vi "HW XML Rx - Write.vi"(0 "String (in)":string, 7 "Parameter Array":T1[](array[typedef])) -> (4 "String (out)":string)   [LabVIEW 2017]
uses:
  Controls/Database_Array.ctl
  Controls/Encoding.ctl
  <userlib>/_OpenG.lib/array/array.llb/Remove Duplicates from 1D Array (I32)__ogtk.vi
  <userlib>/_OpenG.lib/array/array.llb/Filter 1D Array with Scalar (I32)__ogtk.vi
  <userlib>/_OpenG.lib/array/array.llb/Index 1D Array Elements (Variant)__ogtk.vi
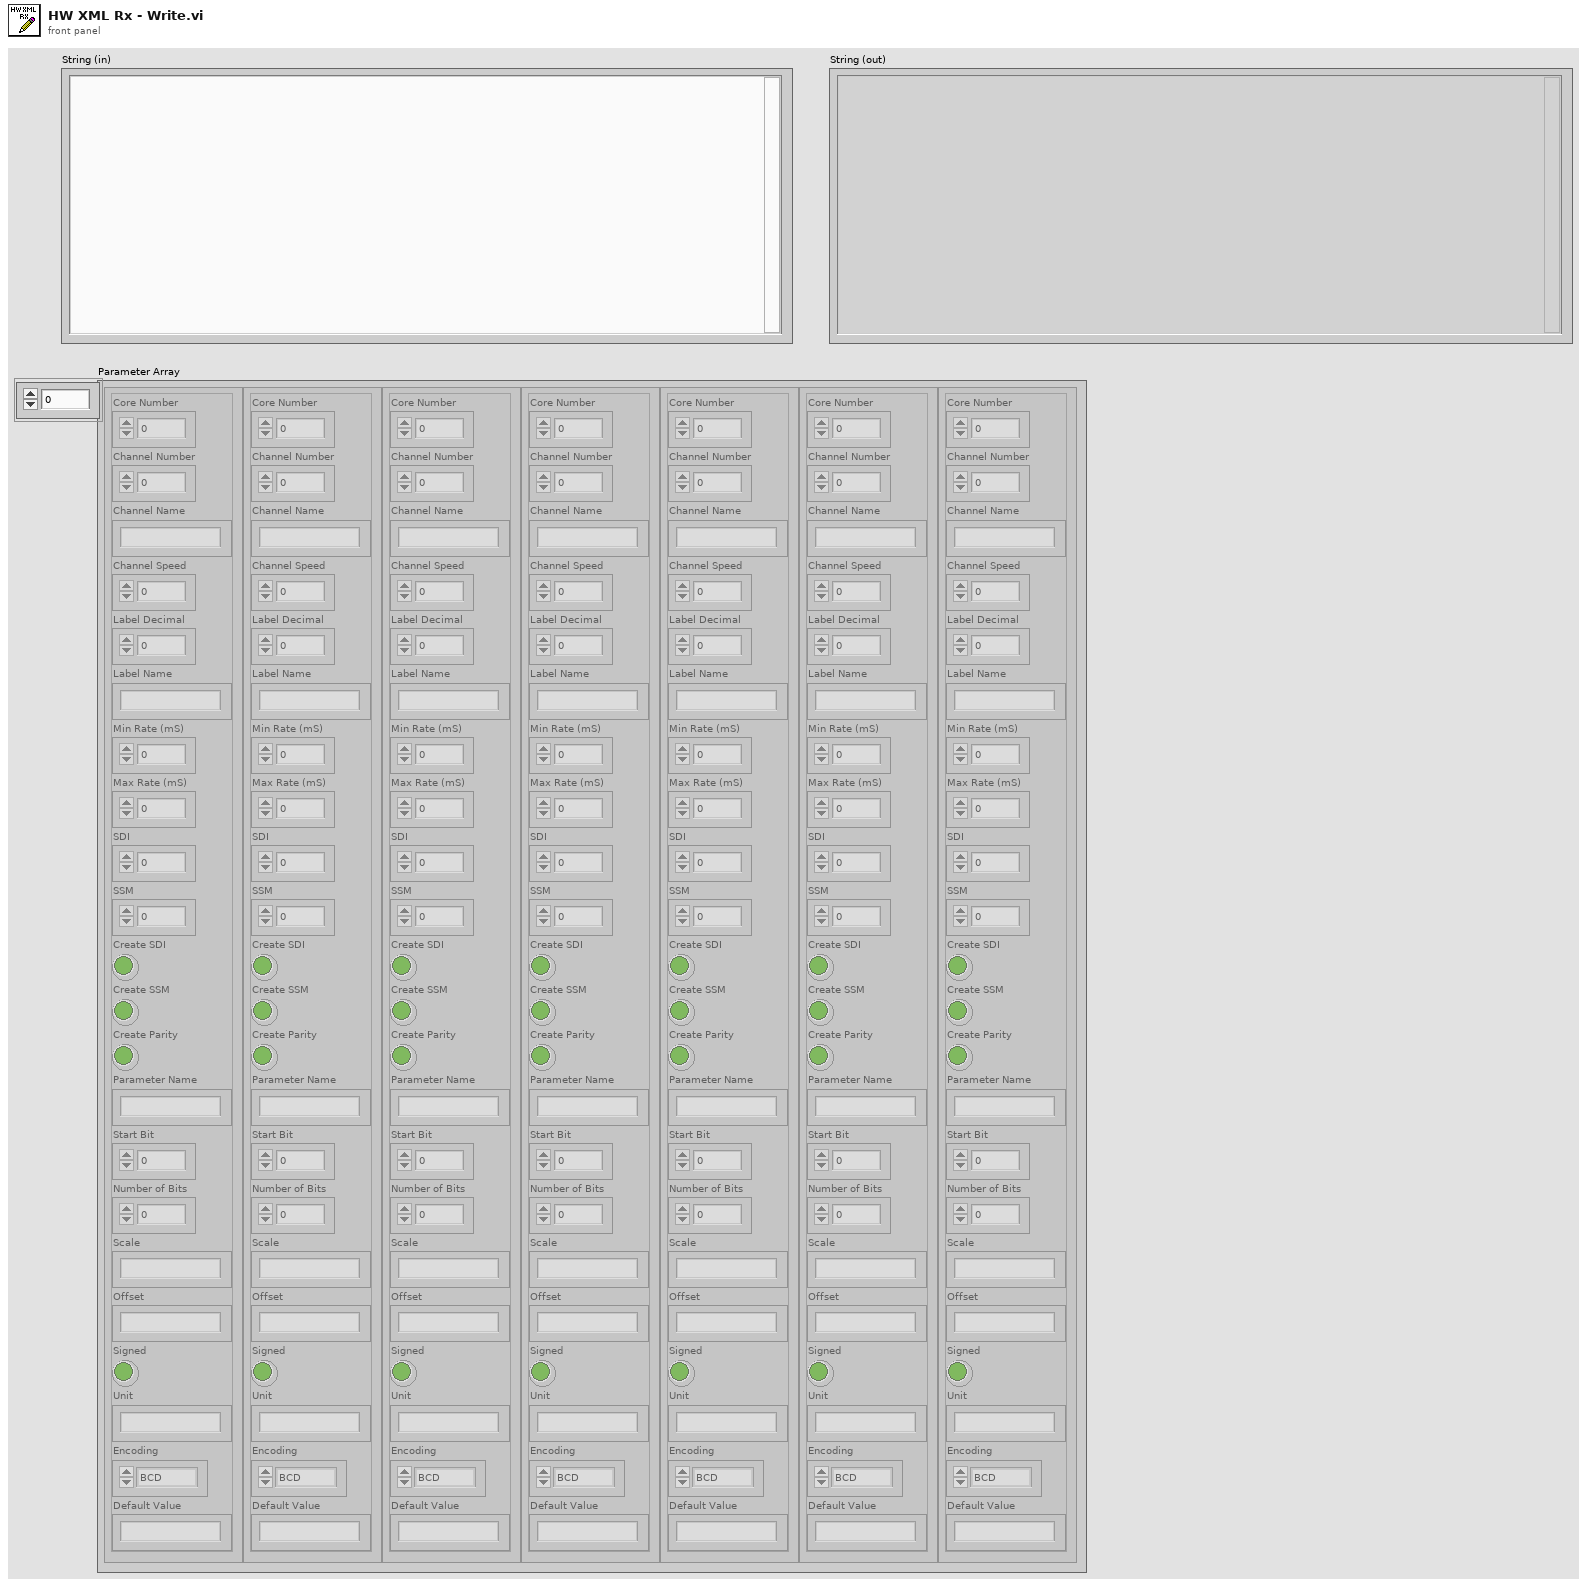
[diagram p1: front panel]
types:
  T1 = typedef "Database_Array.ctl" = cluster{"Core Number":i32, "Channel Number":i32, "Channel Name":string, "Channel Speed":i32, "Label Decimal":i32, "Label Name":string, "Min Rate (mS)":i32, "Max Rate (mS)":i32, "SDI":i32, "SSM":i32, "Create SDI":bool, "Create SSM":bool, "Create Parity":bool, "Parameter Name":string, "Start Bit":i32, "Number of Bits":i32, "Scale":string, "Offset":string, "Signed":bool, "Unit":string, "Encoding":T2, "Default Value":string}
  T2 = typedef "Encoding.ctl" = enum16{"BCD", "BNR", "Discrete"}
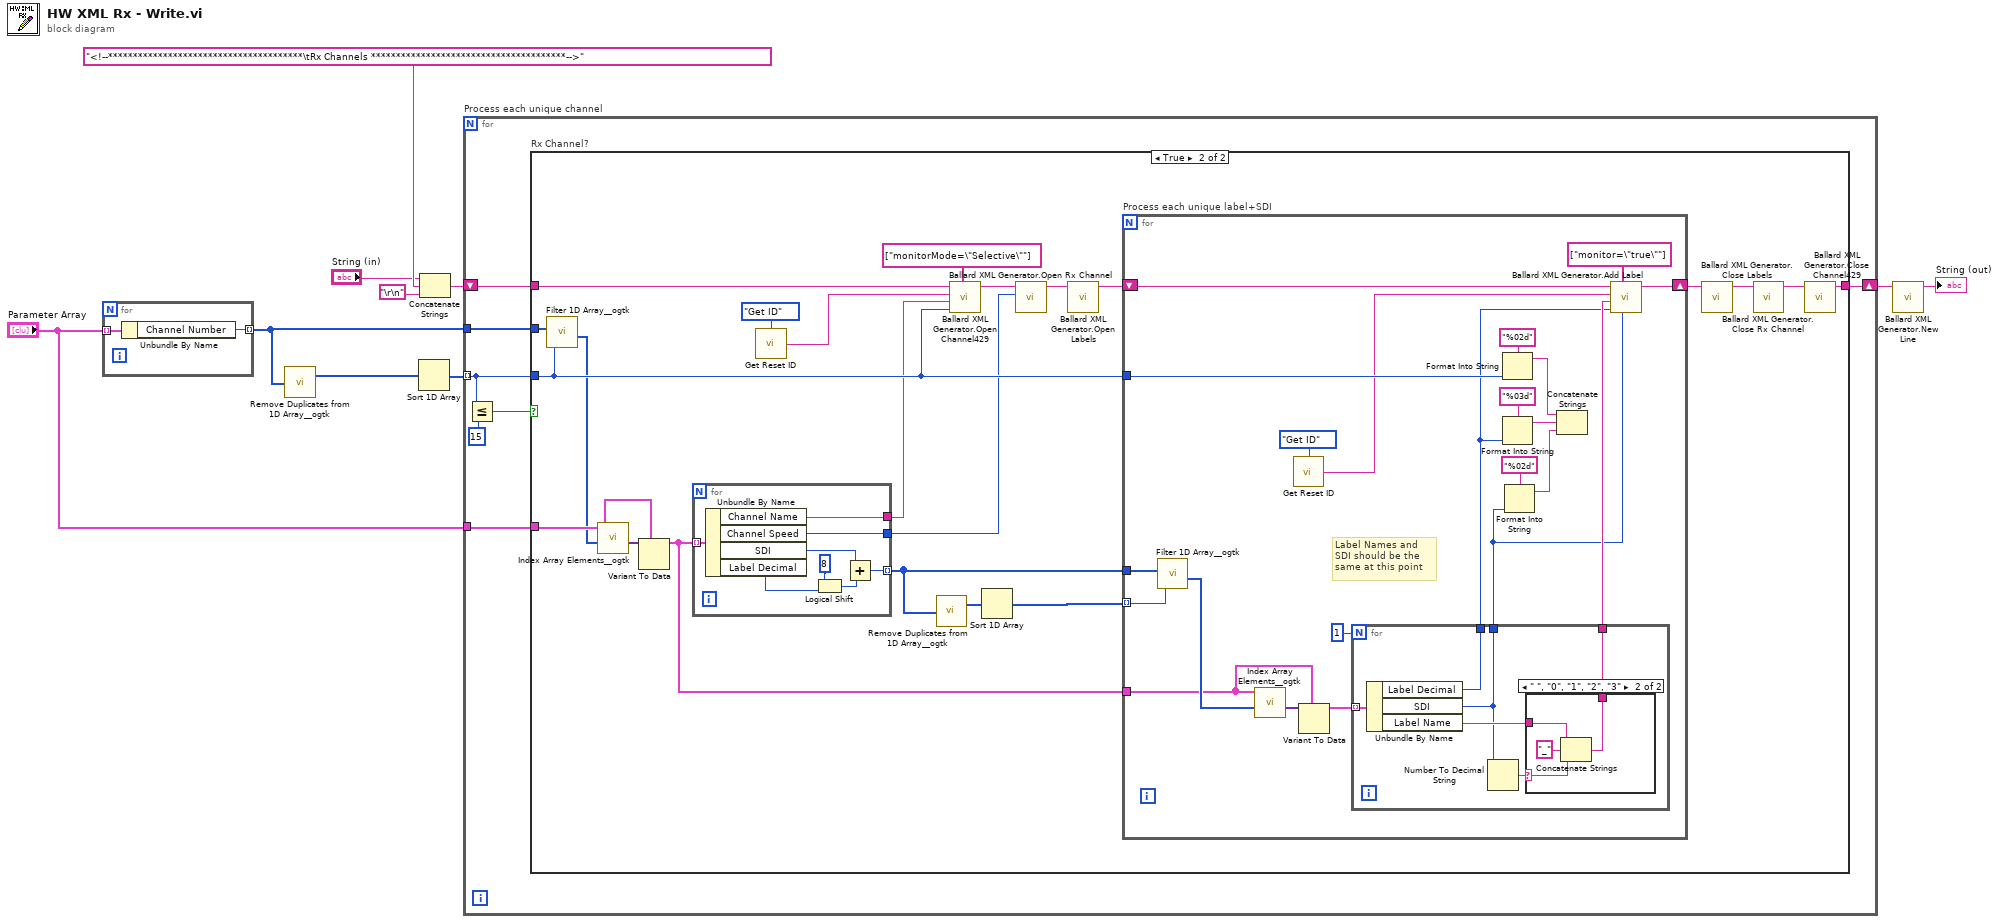
[diagram p0: block diagram]
diagram:
  n1 = for {
    tunnel: [w12] -> w3 mode=indexing
    tunnel: "Parameter Array" -> [w11] mode=indexing
    n2 = Unbundle By Name(w11) -> ("Channel Number"=w12:i32)
  }
  n3 = call-poly <userlib>:"Remove Duplicates from 1D Array__ogtk.vi"("Input Array"=w3) -> ("Output Array"=w9:i32[])  [unwired: 1 out]
  n4 = Sort 1D Array(array=w9) -> (sorted array=w10:i32[])
  n5 = Concatenate Strings("String (in)", "<!--***************************************\tRx Channels ***************************************-->", "\r\n") -> (w6:string)
  n6 = for "Process each unique channel" {
    tunnel: w10 -> [w17] mode=indexing
    shift-right: [w18] -> w1
    shift-left: w6 -> [w19]
    tunnel: w3 -> [w14]
    tunnel: "Parameter Array" -> [w13]
    n7 = Less Or Equal?(x=w17, y=15) -> (x <= y?=w16:bool)
    n8 = case "Rx Channel?" shown="True" w16 {
      tunnel: w19 -> [w20 w40]
      tunnel: [w20 w32] -> w18
      tunnel: w17 -> [_ w31]
      tunnel: w14 -> [_ w30]
      tunnel: w13 -> [_ w28]
      frame False {
      }
      frame True {
        n9 = call-poly <userlib>:"Filter 1D Array__ogtk.vi"("items to filter"=w31, "array"=w30) -> ("filtered item indices"=w26:i32[])  [unwired: 4 in, 1 out]
        n10 = call-poly <userlib>:"Index Array Elements__ogtk.vi"("indices"=w26, "array"=w28) -> ("elements"=w29:variant[])  [unwired: 9 in]
        n11 = Variant To Data(type=w28, Variant=w29) -> (data=w25:T1[])  [unwired: 1 in, 1 out]
        n12 = for {
          tunnel: w25 -> [w50] mode=indexing
          tunnel: [w49] -> w24
          tunnel: [w48] -> w23
          tunnel: [w44] -> w27 mode=indexing
          n13 = Unbundle By Name(w50) -> ("Channel Name"=w49:string, "Channel Speed"=w48:i32, "SDI"=w43:i32, "Label Decimal"=w45:i32)
          n14 = Logical Shift(y=i16 8, x=w45) -> (x << y=w47:i32)
          n15 = Add(x=w43, y=w47) -> (x+y=w44:i32)
        }
        n16 = call "Get Reset ID.vi"("Function"=enum16{"Get ID", "Reset ID"}."Get ID") -> ("ID"=w21:string)  [unwired: 14 in]
        n17 = call-poly <userlib>:"Remove Duplicates from 1D Array__ogtk.vi"("Input Array"=w27) -> ("Output Array"=w42:i32[])  [unwired: 1 out]
        n18 = call "Ballard XML Generator.Open Channel429.vi"("other params"=string[] ["monitorMode=\"Selective\""], "hardware channel"=w31, "name"=w24, "id"=w21, "string in"=w40) -> ("string out"=w37:string)  [unwired: 6 in]
        n19 = Sort 1D Array(array=w42) -> (sorted array=w41:i32[])
        n20 = call "Ballard XML Generator.Open Rx Channel.vi"("speedKHz"=w23, "string in"=w37) -> ("string out"=w38:string)  [unwired: 9 in]
        n21 = call "Ballard XML Generator.Open Labels.vi"("string in"=w38) -> ("string out"=w36:string)  [unwired: 10 in]
        n22 = for "Process each unique label+SDI" {
          tunnel: w41 -> [w66] mode=indexing
          tunnel: w27 -> [w72]
          shift-right: [w69] -> w35
          shift-left: w36 -> [w70]
          tunnel: w31 -> [w65]
          tunnel: w25 -> [w60]
          # "Label Names and SDI should be the same at this point"
          n23 = call-poly <userlib>:"Filter 1D Array__ogtk.vi"("items to filter"=w66, "array"=w72) -> ("filtered item indices"=w62:i32[])  [unwired: 4 in, 1 out]
          n24 = call-poly <userlib>:"Index Array Elements__ogtk.vi"("indices"=w62, "array"=w60) -> ("elements"=w61:variant[])  [unwired: 9 in]
          n25 = call "Get Reset ID.vi"("Function"=enum16{"Get ID", "Reset ID"}."Get ID") -> ("ID"=w51:string)  [unwired: 14 in]
          n26 = Variant To Data(type=w60, Variant=w61) -> (data=w59:T1[])  [unwired: 1 in, 1 out]
          n27 = for {
            N: 1 -> [_]
            tunnel: w59 -> [w78] mode=indexing
            tunnel: [w76] -> w58
            tunnel: [w77] -> w57
            tunnel: [w73] -> w53
            n28 = Unbundle By Name(w78) -> ("Label Decimal"=w77:i32, "SDI"=w73:i32, "Label Name"=w74:string)
            n29 = Number To Decimal String(number=w73) -> (decimal integer string=w75:string)  [unwired: 1 in]
            n30 = case shown="\" \", \"0\", \"1\", \"2\", \"3\"" w75 {
              selector: w75 -> [_ w80]
              tunnel: w74 -> [w79 w83]
              tunnel: [w79 w81] -> w76
              frame "False", Default {
              }
              frame " ", "0", "1", "2", "3" {
                n31 = Concatenate Strings(w83, "_" ("string"), w80) -> (w81:string)
              }
            }
          }
          n32 = Format Into String(format string="%02d", w65) -> (resulting string=w64:string)  [unwired: 2 in, 1 out]
          n33 = Format Into String(format string="%03d", w57) -> (resulting string=w63:string)  [unwired: 2 in, 1 out]
          n34 = Format Into String(format string="%02d", w53) -> (resulting string=w54:string)  [unwired: 2 in, 1 out]
          n35 = Concatenate Strings(w64, w63, w54) -> ()  [unwired: 1 out]
          n36 = call "Ballard XML Generator.Add Label.vi"("SDI"=w53, "other params"=string[] ["monitor=\"true\""], "label decimal"=w57, "name"=w58, "id"=w51, "string in"=w70) -> ("string out"=w69:string)  [unwired: 5 in]
        }
        n37 = call "Ballard XML Generator.Close Labels.vi"("string in"=w35) -> ("string out"=w34:string)  [unwired: 10 in]
        n38 = call "Ballard XML Generator.Close Rx Channel.vi"("string in"=w34) -> ("string out"=w33:string)  [unwired: 10 in]
        n39 = call "Ballard XML Generator.Close Channel429.vi"("string in"=w33) -> ("string out"=w32:string)  [unwired: 10 in]
      }
    }
  }
  n40 = call "Ballard XML Generator.New Line.vi"("string in"=w1) -> ("string out"=→"String (out)":string)  [unwired: 10 in]
